vi "env-toolkit-ui.vi"() -> ()   [LabVIEW 2025]
doc: "Environment Toolkit for TestStand - Graphical User Interface"
uses:
  TSDiscovery/TSDiscovery.lvclass
  C:/Users/juanj/Documents/hasbun_wood_engineering/github/Environment-Toolkit-for-TestStand/src/TSDiscovery/TSDiscovery.lvclass
  C:/Users/juanj/Documents/hasbun_wood_engineering/github/Environment-Toolkit-for-TestStand/src/ITSDiscovery/ITSDiscovery.lvclass
  TSDiscovery Mock/TSDiscovery Mock.lvclass
  C:/Users/juanj/Documents/hasbun_wood_engineering/github/Environment-Toolkit-for-TestStand/src/TSDiscovery Mock/TSDiscovery Mock.lvclass
  Process Executor/Process Executor.lvclass
  C:/Users/juanj/Documents/hasbun_wood_engineering/github/Environment-Toolkit-for-TestStand/src/Process Executor/Process Executor.lvclass
  C:/Users/juanj/Documents/hasbun_wood_engineering/github/Environment-Toolkit-for-TestStand/src/IProcess Executor/IProcess Executor.lvclass
  Type Definitions/UI State--enum.ctl
  Libraries/TS Environment Manager/TS Environment Manager.lvlib
  Type Definitions/UI Data--cluster.ctl
  Type Definitions/Architecture--enum.ctl
  Type Definitions/Profile--cluster.ctl
  Type Definitions/TSInstall--cluster.ctl
  <vilib>/Utility/miscctls.llb/LVRectTypeDef.ctl
  <vilib>/Utility/miscctls.llb/LVPointTypeDef.ctl
  Type Definitions/Progress Display--enum.ctl
  Type Definitions/Execution Plan--cluster.ctl
  <vilib>/Platform/browser.llb/Open URL in Default Browser (string).vi
  ITSDiscovery/ITSDiscovery.lvclass
  IProcess Executor/IProcess Executor.lvclass
panel:
  in  "Open":bool
  out "Progress Display String":string
  in  "License":bool
  in  "Clear Environment":bool
  in  "Progress Display":T1
  in  "New Profiles File":path
  in  "Environment (Profile Mgt)":path caption="Environment"
  out "Environment (Launch)":path caption="Environment"
  in  "Hyperlink HWE":bool
  in  "Third Party Licenses":bool
  in  "Launch":bool
  in  "Set File":bool
  in  "Delete Profile":bool
  in  "Add Profile":bool
  in  "New Profile Name":string
  in  "Profiles":i32(listbox)
  in  "Installations":i32(listbox)
  out "Profiles File":path
  # "Hidden elements"
  # "Profile Management"
  # "Launch"
  # "This software is released under the MIT License\nCopyright (c) 2026 Juan Jose Hasbun Wood"
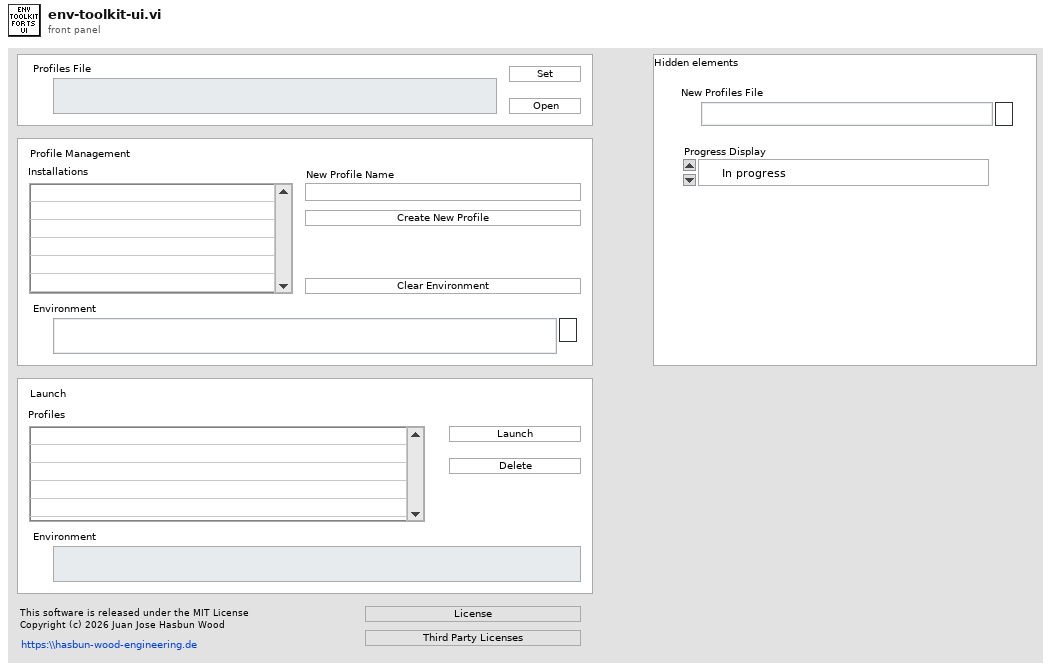
[diagram p1: front panel]
types:
  T1 = typedef "Progress Display--enum.ctl" = enum16{"     In progress", "     In progress.", "     In progress..", "     In progress..."}
  T2 = typedef "UI Data--cluster.ctl" = cluster{"Profiles":T3[], "Installations":T5[], "Event Structure Timeout":i32, "IProcess Executor.lvclass":refnum<class "IProcess Executor.lvclass">, "ITSDiscovery.lvclass":refnum<class "ITSDiscovery.lvclass">}
  T3 = typedef "Profile--cluster.ctl" = cluster{"Name":string, "Version":string, "Architecture":T4, "Environment":path}
  T4 = typedef "Architecture--enum.ctl" = enum16{"32bit", "64bit"}
  T5 = typedef "TSInstall--cluster.ctl" = cluster{"Version":string, "Architecture":T4, "Version Key":string, "ID":string}
  T6 = typedef "UI State--enum.ctl" = enum16{"Init", "Idle", "Add", "Delete", "Launch SeqEdit", "Error", "Exit", "License", "Update Profiles", "Update Installations", "Set File", "Start In Progress", "Stop In Progress", "Activate Version", "Third Party Licenses"}
  T7 = typedef "TS Environment Manager.lvlib/Broadcast Events--cluster.ctl" = cluster{"Module Did Init":refnum<user-event>, "Status Updated":refnum<user-event>, "Error Reported":refnum<user-event>, "Module Did Stop":refnum<user-event>, "Update Module Execution Status":refnum<user-event>, "Version Activated":refnum<user-event>, "Launched SeqEdit":refnum<user-event>}
  T8 = typedef "LVPointTypeDef.ctl" = cluster{"Horizontal":i16, "Vertical":i16}
  T9 = typedef "Execution Plan--cluster.ctl" = cluster{"Exe Path":path, "Args":string[], "Timeout":i32}
  T10 = typedef "LVRectTypeDef.ctl" = cluster{"Left":i16, "Top":i16, "Right":i16, "Bottom":i16}
  T11 = enum8{"Enabled", "Disabled", "Disabled and Grayed Out"}
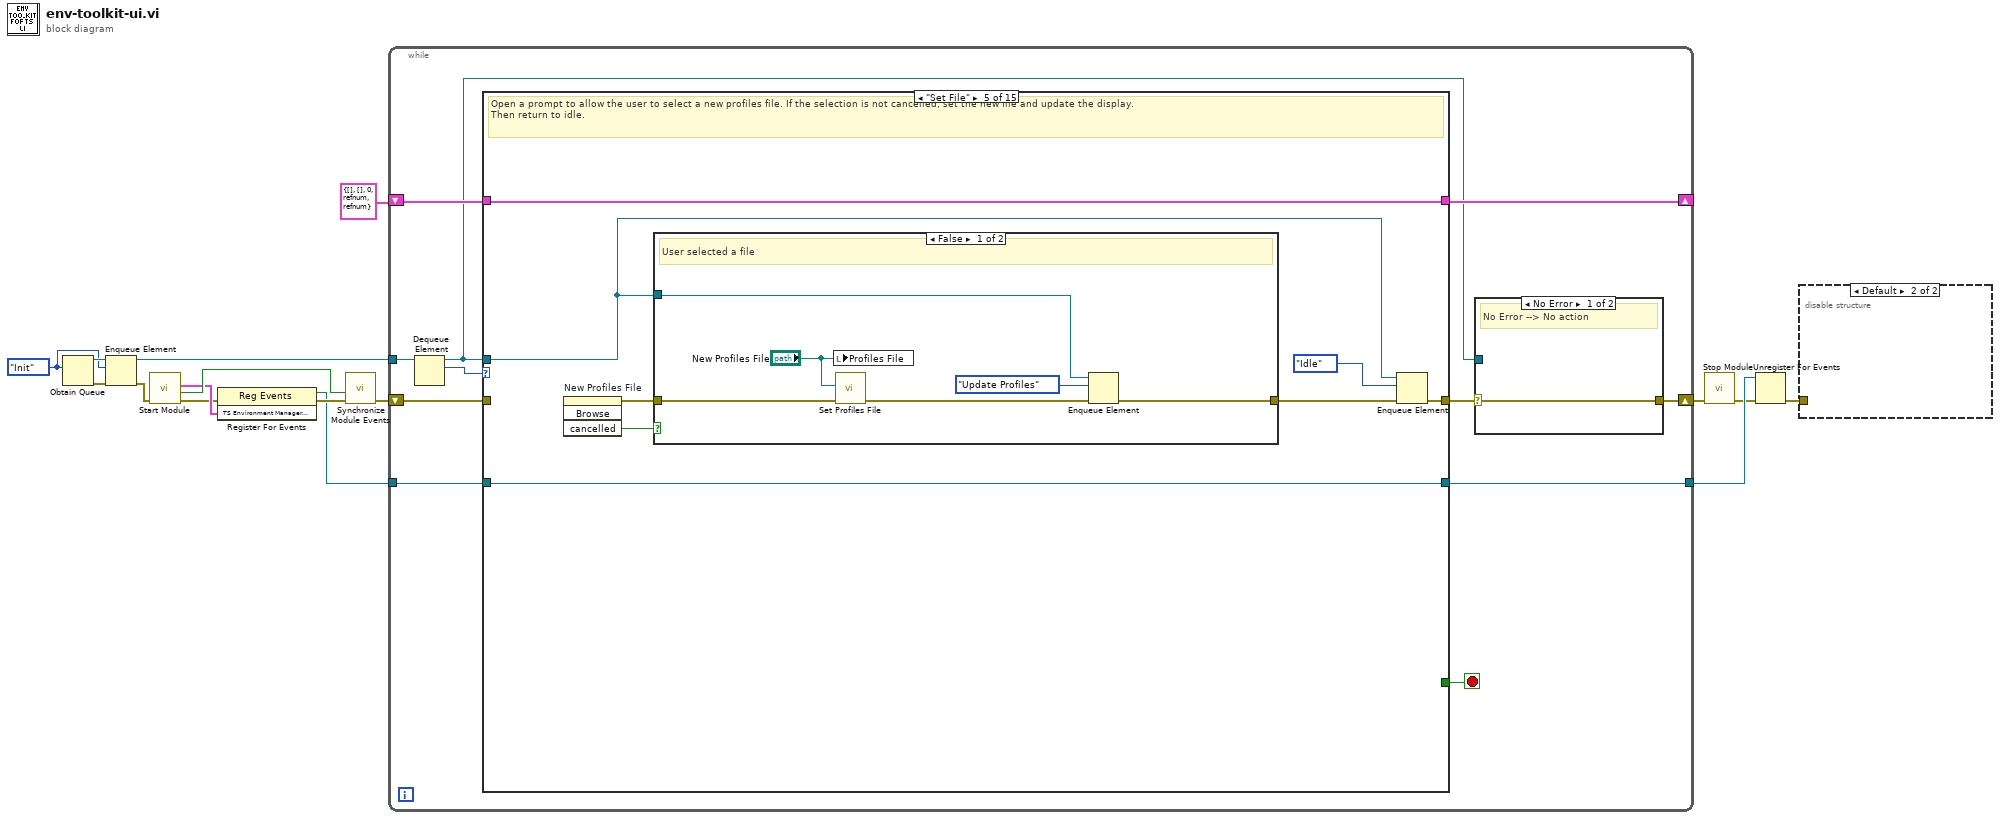
[diagram p0: block diagram]
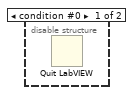
[diagram p2: hidden frame]
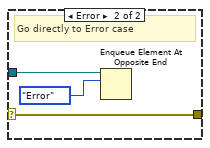
[diagram p3: hidden frame]
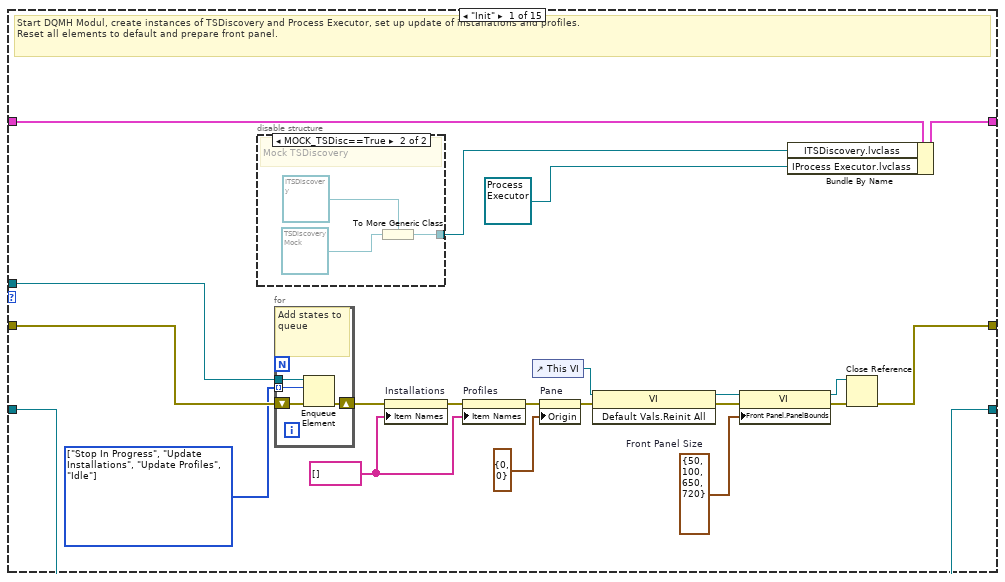
[diagram p4: hidden frame]
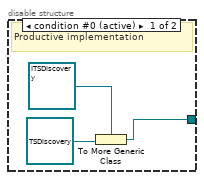
[diagram p5: hidden frame]
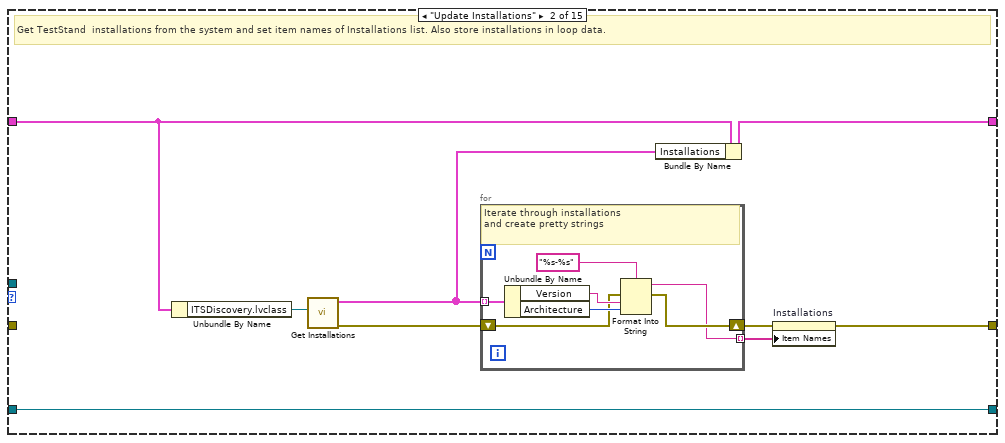
[diagram p6: hidden frame]
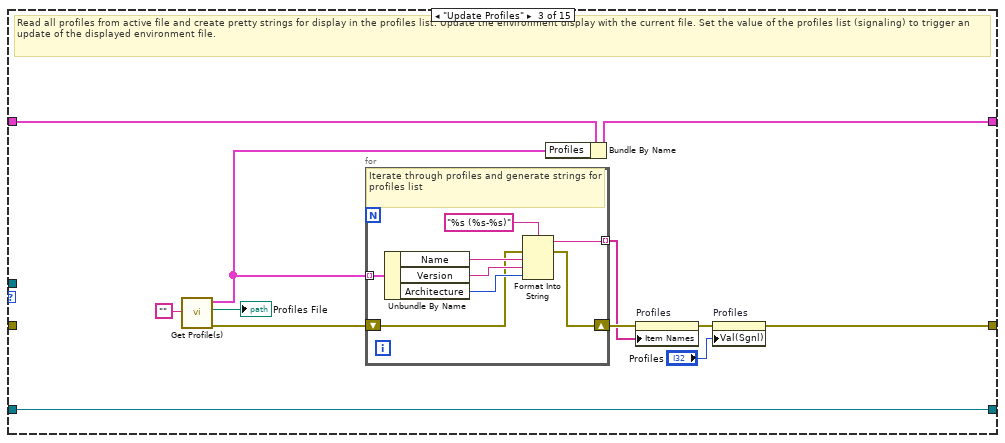
[diagram p7: hidden frame]
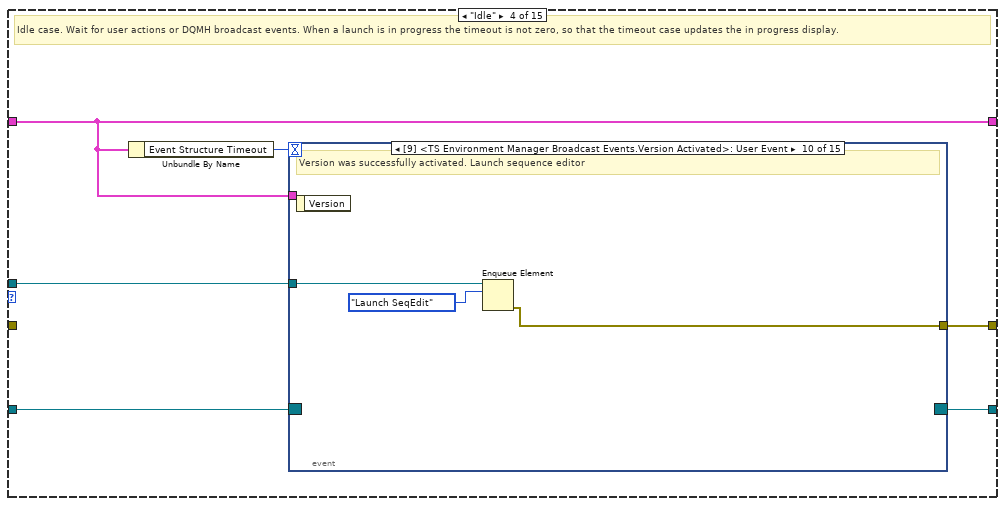
[diagram p8: hidden frame]
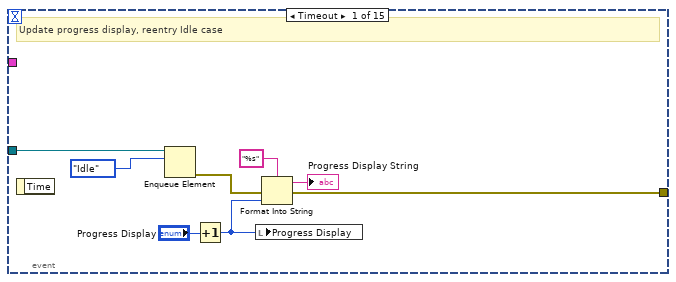
[diagram p9: hidden frame]
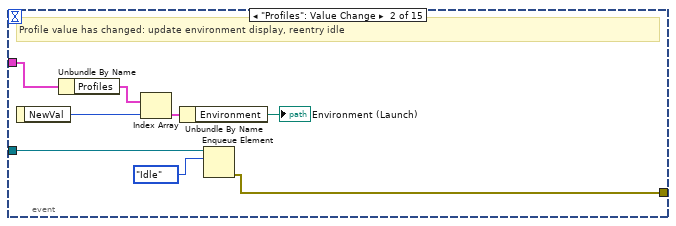
[diagram p10: hidden frame]
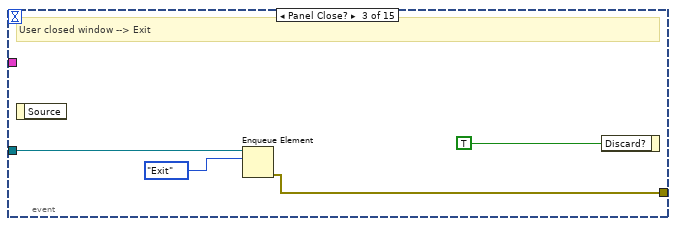
[diagram p11: hidden frame]
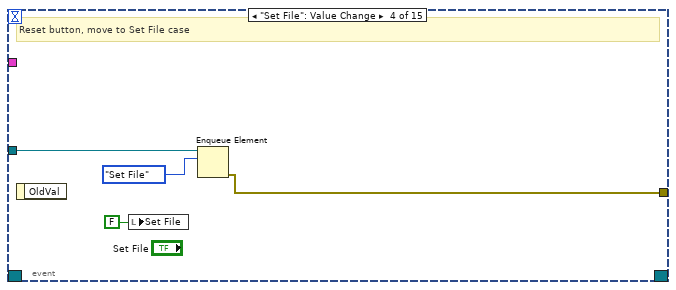
[diagram p12: hidden frame]
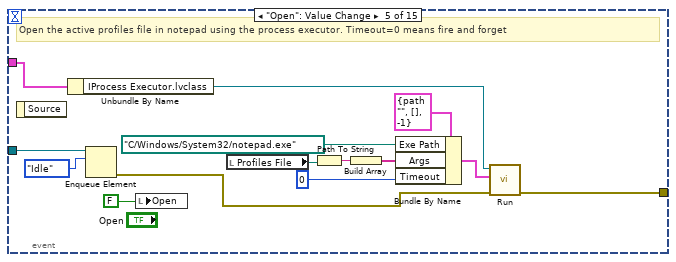
[diagram p13: hidden frame]
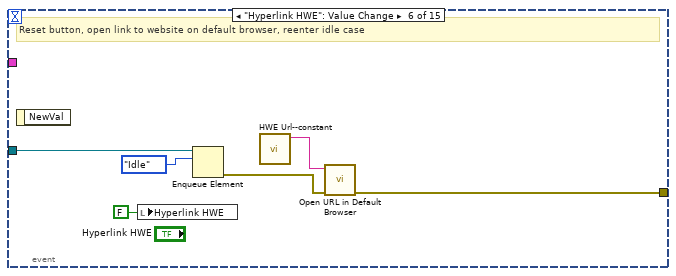
[diagram p14: hidden frame]
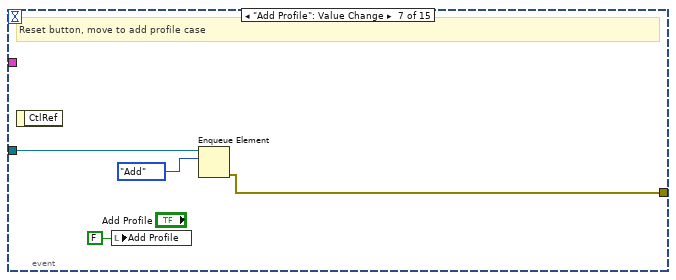
[diagram p15: hidden frame]
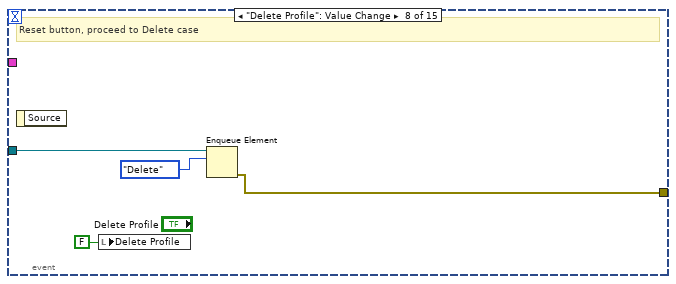
[diagram p16: hidden frame]
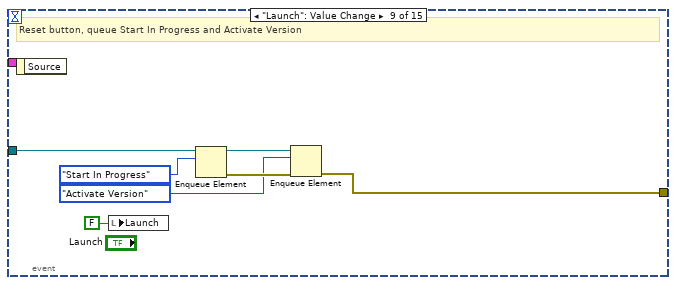
[diagram p17: hidden frame]
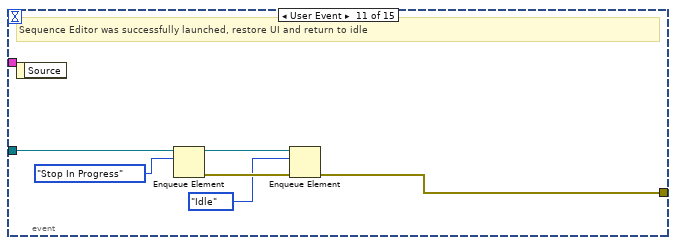
[diagram p18: hidden frame]
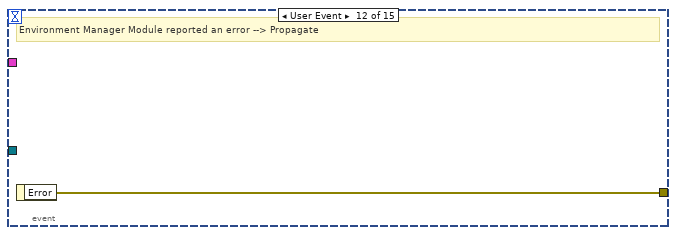
[diagram p19: hidden frame]
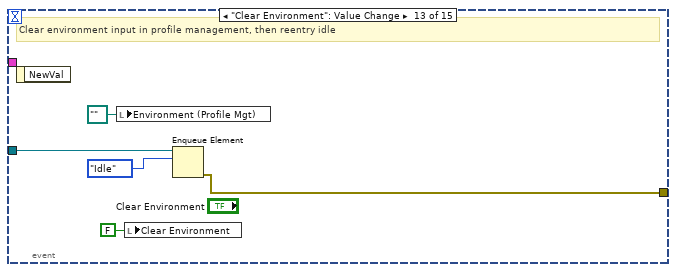
[diagram p20: hidden frame]
diagram:
  w14 = UI_State--enum."Init"
  n1 = Obtain Queue(element data type=w14) -> (queue out=w16:refnum<queue>, error out=w15:errorcluster)  [unwired: 4 in, 1 out]
  n2 = Enqueue Element(queue=w16, element=w14, error in (no error)=w15) -> (queue out=w13:refnum<queue>, error out=w7:errorcluster)  [unwired: 1 in, 1 out]
  n3 = call "Start Module.vi"("error in"=w7) -> ("error out"=w9:errorcluster, "Wait for Event Sync?"=w11:bool, "TS Environment Manager Broadcast Events"=w10:T7)  [unwired: 6 in, 2 out]
  n4 = register-events(error in=w9, w10) -> (reference out=w5:refnum<event-registration>, error out=w8:errorcluster)  [unwired: 1 in]
  n5 = call "Synchronize Module Events.vi"("error in"=w8, "Wait for Event Sync?"=w11) -> ("error out"=w6:errorcluster)  [unwired: 9 in]
  n6 = while {
    tunnel: w13 -> [w27]
    shift-right: [w22] -> w2
    shift-left: w6 -> [w17]
    shift-right: [w24] -> _
    shift-left: T2 {"Profiles"=[], "Installations"=[], "Event Structure Timeout"=0, "IProcess Executor.lvclass"=refnum, "ITSDiscovery.lvclass"=refnum} ("UI Data") -> [w25]
    tunnel: w5 -> [w19]
    tunnel: [w18] -> w3
    stop <- w20 stop-if-true
    n7 = Dequeue Element(queue=w27) -> (queue out=w21:refnum<queue>, element=w26:T6)  [unwired: 2 in, 2 out]
    n8 = case shown="\"Set File\"" w26 {
      tunnel: w21 -> [w49 _ _ w104 w190 w208 _ w235 w252 w262 w280 w294 w304 _ _]
      tunnel: w17 -> [w48 _ _ _ _ w205 _ _ _ _ _ _ _ _ _]
      tunnel: w25 -> [w52 w65 w85 w99 w187 w202 w219 w225 w242 w272 w286 w297 w314 w325 w347]
      tunnel: [w50 w66 w86 w99 w187 w202 w219 w225 w242 w272 w286 w297 w314 w326 w348] -> w24
      tunnel: [w32 w67 w81 w103 w191 w207 w216 w222 w237 w255 w278 w295 w308 w327 w349] -> w23
      tunnel: [_ _ _ _ _ _ TRUE _ _ _ _ _ _ _ _] -> w20
      tunnel: w19 -> [w34 w63 w79 w102 w188 w206 w218 w236 w253 w259 w277 w291 w305 w323 w345]
      tunnel: [w34 w63 w79 w100 w188 w206 w218 w236 w253 w259 w277 w291 w305 w323 w345] -> w18
      frame "Init" {
        w41 = T10 {"Left"=50, "Top"=100, "Right"=650, "Bottom"=720}  # Front Panel Size
        w45 = string[] [] ("Item Names")
        w47 = T6[] [enum."Stop In Progress", enum."Update Installations", enum."Update Profiles", enum."Idle"] items=["Init", "Idle", "Add", "Delete", "Launch SeqEdit", "Error", "Exit", "License", "Update Profiles", "Update Installations", "Set File", "Start In Progress", "Stop In Progress", "Activate Version", "Third Party Licenses"]
        # "Start DQMH Modul, create instances of TSDiscovery and Process Executor, set up update of installations and profiles.\nReset all elements to default and prepare front panel."
        n9 = disable-structure shown="MOCK_TSDisc==True" {
          disable-tunnel: [w53 w56] -> w33
          frame condition #0 (active) {
            # "Productive implementation"
            n10 = To More Generic Class(target class=refnum<class "ITSDiscovery.lvclass"> refnum ("ITSDiscovery.lvclass"), reference=refnum<class "TSDiscovery.lvclass"> refnum ("TSDiscovery.lvclass")) -> (generic class reference=w53:refnum<class "ITSDiscovery.lvclass">)
          }
          frame condition #1 {
            # "Mock TSDiscovery"
            n11 = To More Generic Class(target class=refnum<class "ITSDiscovery.lvclass"> refnum ("ITSDiscovery.lvclass"), reference=refnum<class "TSDiscovery Mock.lvclass"> refnum ("TSDiscovery Mock.lvclass")) -> (generic class reference=w56:refnum<class "ITSDiscovery.lvclass">)
          }
        }
        n12 = for {
          tunnel: w49 -> [w62]
          tunnel: w47 -> [w60] mode=indexing
          shift-right: [w59] -> w36
          shift-left: w48 -> [w61]
          # "Add states to queue"
          n13 = Enqueue Element(queue=w62, element=w60, error in (no error)=w61) -> (error out=w59:errorcluster)  [unwired: 1 in, 2 out]
        }
        n14 = property on="Installations" class="LstBox (strict)"(error in=w36, "Item Names"=w45) -> (error out=w46:errorcluster)  [unwired: 1 in, 1 out]
        n15 = property on="Profiles" class="LstBox (strict)"(error in=w46, "Item Names"=w45) -> (error out=w44:errorcluster)  [unwired: 1 in, 1 out]
        n16 = control-ref of="This VI"() -> (w42:refnum<vi>)
        n17 = property on="Pane" class="Pane"(error in=w44, "Origin"=T8 {"Horizontal"=0, "Vertical"=0}) -> (error out=w43:errorcluster)  [unwired: 1 in, 1 out]
        n18 = invoke on="Invoke Node" class="VI" method="Default Vals.Reinit All"(reference=w42, error in=w43) -> (reference out=w40:refnum<vi>, error out=w39:errorcluster)  [unwired: 1 in, 1 out]
        n19 = property on="Property Node" class="VI"(reference=w40, error in=w39, "Front Panel.PanelBounds"=w41) -> (reference out=w38:refnum<vi>, error out=w37:errorcluster)
        n20 = Bundle By Name(cluster=w52, "ITSDiscovery.lvclass"=w33, "IProcess Executor.lvclass"=refnum<class "Process Executor.lvclass"> refnum ("Process Executor.lvclass")) -> (w50:T2)
        n21 = Close Reference(reference=w38, error in (no error)=w37) -> (error out=w32:errorcluster)
      }
      frame "Update Installations" {
        # "Get TestStand  installations from the system and set item names of Installations list. Also store installations in loop data."
        n22 = Unbundle By Name(w65) -> ("ITSDiscovery.lvclass"=w68:refnum<class "ITSDiscovery.lvclass">)
        n23 = call "Get Installations.vi"("ITSDiscovery.lvclass"=w68) -> ("error out"=w71:errorcluster, "Installations"=w64:T5[])  [unwired: 8 in, 1 out]
        n24 = for {
          tunnel: w64 -> [w78] mode=indexing
          shift-right: [w73] -> w69
          shift-left: w71 -> [w74]
          tunnel: [w72] -> w70 mode=indexing
          # "Iterate through installations\nand create pretty strings"
          n25 = Unbundle By Name(w78) -> ("Version"=w76:string, "Architecture"=w75:T4)
          n26 = Format Into String(format string="%s-%s", error in=w74, w76, w75) -> (resulting string=w72:string, error out=w73:errorcluster)  [unwired: 1 in]
        }
        n27 = Bundle By Name(cluster=w65, "Installations"=w64) -> (w66:T2)
        n28 = property on="Installations" class="LstBox (strict)"(error in=w69, "Item Names"=w70) -> (error out=w67:errorcluster)  [unwired: 1 in, 1 out]
      }
      frame "Update Profiles" {
        # "Read all profiles from active file and create pretty strings for display in the profiles list. Update the environment display with the current file. Set the value of the profiles list (signaling) to trigger an update of the displayed environment file."
        n29 = call "Get Profile(s).vi"("Name"="" ("Empty String Constant")) -> ("error out"=w89:errorcluster, "File"=→"Profiles File":path, "Profile(s)"=w84:T3[])  [unwired: 7 in, 1 out]
        n30 = for {
          tunnel: w84 -> [w98] mode=indexing
          shift-right: [w92] -> w88
          shift-left: w89 -> [w93]
          tunnel: [w91] -> w87 mode=indexing
          # "Iterate through profiles and generate strings for profiles list"
          n31 = Unbundle By Name(w98) -> ("Name"=w96:string, "Version"=w95:string, "Architecture"=w94:T4)
          n32 = Format Into String(format string="%s (%s-%s)", error in=w93, w96, w95, w94) -> (resulting string=w91:string, error out=w92:errorcluster)  [unwired: 1 in]
        }
        n33 = Bundle By Name(cluster=w85, "Profiles"=w84) -> (w86:T2)
        n34 = property on="Profiles" class="LstBox (strict)"(error in=w88, "Item Names"=w87) -> (error out=w82:errorcluster)  [unwired: 1 in, 1 out]
        n35 = property on="Profiles" class="LstBox (strict)"(error in=w82, "Val(Sgnl)"="Profiles") -> (error out=w81:errorcluster)  [unwired: 1 in, 1 out]
      }
      frame "Idle" {
        # "Idle case. Wait for user actions or DQMH broadcast events. When a launch is in progress the timeout is not zero, so that the timeout case updates the in progress display."
        n36 = Unbundle By Name(w99) -> ("Event Structure Timeout"=w101:i32)
        n37 = event shown="[9] <TS Environment Manager Broadcast Events.Version Activated>: User Event" {
          selector: w102 -> [_ _ _ _ _ _ _ _ _ _ _ _ _ _ _]
          dyn-events: [_ _ _ _ _ _ _ _ _ _ _ _ _ _ _] -> w100
          timeout: w101 -> [_ _ _ _ _ _ _ _ _ _ _ _ _ _ _]
          tunnel: w99 -> [_ w113 _ _ w129 _ _ _ _ _ _ _ _ _ _]
          tunnel: w104 -> [w107 w116 w123 w128 w141 w145 w152 w156 w162 w166 w172 _ w176 w181 w186]
          tunnel: [w108 w115 w121 w126 w131 w147 w151 w155 w160 w165 w170 w173 w174 w180 w185] -> w103
          event Timeout {
            # "Update progress display, reentry Idle case"
            n38 = event-data() -> ()  [unwired: 1 in, 1 out]
            n39 = Enqueue Element(queue=w107, element=UI_State--enum."Idle") -> (error out=w105:errorcluster)  [unwired: 2 in, 2 out]
            n40 = Increment(x="Progress Display") -> (x+1=w111:T1)
            n41 = local write "Progress Display"(w111) -> ()
            n42 = Format Into String(format string="%s", error in=w105, w111) -> (resulting string=→"Progress Display String":string, error out=w108:errorcluster)  [unwired: 1 in]
          }
          event "Profiles": Value Change {
            # "Profile value has changed: update environment display, reentry idle"
            n43 = event-data() -> ("NewVal"=w119:i32)  [unwired: 1 in]
            n44 = Unbundle By Name(w113) -> ("Profiles"=w120:T3[])
            n45 = Index Array(array=w120, index=w119) -> (element=w118:T3)
            n46 = Unbundle By Name(w118) -> ("Environment"=→"Environment (Launch)":path)
            n47 = Enqueue Element(queue=w116, element=UI_State--enum."Idle") -> (error out=w115:errorcluster)  [unwired: 2 in, 2 out]
          }
          event Panel Close? {
            # "User closed window --> Exit"
            n48 = event-data() -> ()  [unwired: 1 in, 1 out]
            n49 = Enqueue Element(queue=w123, element=UI_State--enum."Exit") -> (error out=w121:errorcluster)  [unwired: 2 in, 2 out]
            n50 = event-data ("Event Filter Node")("Discard?"=TRUE) -> ()  [unwired: 1 in, 1 out]
          }
          event "Set File": Value Change {
            # "Reset button, move to Set File case"
            n51 = event-data() -> ()  [unwired: 1 in, 1 out]
            n52 = local write "Set File"(FALSE ("Set File")) -> ()
            n53 = Enqueue Element(queue=w128, element=UI_State--enum."Set File") -> (error out=w126:errorcluster)  [unwired: 2 in, 2 out]
          }
          event "Open": Value Change {
            # "Open the active profiles file in notepad using the process executor. Timeout=0 means fire and forget"
            n54 = event-data() -> ()  [unwired: 1 in, 1 out]
            n55 = Unbundle By Name(w129) -> ("IProcess Executor.lvclass"=w133:refnum<class "IProcess Executor.lvclass">)
            n56 = Enqueue Element(queue=w141, element=UI_State--enum."Idle") -> (error out=w130:errorcluster)  [unwired: 2 in, 2 out]
            n57 = local write "Open"(FALSE ("Open")) -> ()
            n58 = local read "Profiles File"() -> (w137:path)
            n59 = Path To String(path=w137) -> (string=w136:string)
            n60 = Build Array(w136) -> (w135:string[])
            n61 = Bundle By Name(cluster=T9 {"Exe Path"=path "", "Args"=[], "Timeout"=-1} ("Execution Plan"), "Exe Path"=path "C:/Windows/System32/notepad.exe", "Args"=w135, "Timeout"=0) -> (w132:T9)
            n62 = call-dynamic "Run.vi"("error in"=w130, "Execution Plan"=w132, "IProcess Executor in"=w133) -> ("error out"=w131:errorcluster)  [unwired: 7 in, 1 out]
          }
          event "Hyperlink HWE": Value Change {
            # "Reset button, open link to website on default browser, reenter idle case"
            n63 = event-data() -> ()  [unwired: 1 in, 1 out]
            n64 = local write "Hyperlink HWE"(FALSE ("Hyperlink HWE")) -> ()
            n65 = Enqueue Element(queue=w145, element=UI_State--enum."Idle") -> (error out=w143:errorcluster)  [unwired: 2 in, 2 out]
            n66 = call "HWE Url--constant.vi"() -> ("url"=w148:string)  [unwired: 11 in]
            n67 = call-poly <vilib>:"Open URL in Default Browser.vi"("error in (no error)"=w143, "URL"=w148) -> ("error out"=w147:errorcluster)  [unwired: 4 in, 1 out]
          }
          event "Add Profile": Value Change {
            # "Reset button, move to add profile case"
            n68 = event-data() -> ()  [unwired: 1 in, 1 out]
            n69 = local write "Add Profile"(FALSE ("Add Profile")) -> ()
            n70 = Enqueue Element(queue=w152, element=UI_State--enum."Add") -> (error out=w151:errorcluster)  [unwired: 2 in, 2 out]
          }
          event "Delete Profile": Value Change {
            # "Reset button, proceed to Delete case"
            n71 = event-data() -> ()  [unwired: 1 in, 1 out]
            n72 = local write "Delete Profile"(FALSE ("Delete Profile")) -> ()
            n73 = Enqueue Element(queue=w156, element=UI_State--enum."Delete") -> (error out=w155:errorcluster)  [unwired: 2 in, 2 out]
          }
          event "Launch": Value Change {
            # "Reset button, queue Start In Progress and Activate Version"
            n74 = event-data() -> ()  [unwired: 1 in, 1 out]
            n75 = local write "Launch"(FALSE ("Launch")) -> ()
            n76 = Enqueue Element(queue=w162, element=UI_State--enum."Start In Progress") -> (queue out=w157:refnum<queue>, error out=w159:errorcluster)  [unwired: 2 in, 1 out]
            n77 = Enqueue Element(queue=w157, element=UI_State--enum."Activate Version", error in (no error)=w159) -> (error out=w160:errorcluster)  [unwired: 1 in, 2 out]
          }
          event User Event {
            # "Version was successfully activated. Launch sequence editor"
            n78 = event-data() -> ()  [unwired: 1 in, 1 out]
            n79 = Enqueue Element(queue=w166, element=UI_State--enum."Launch SeqEdit") -> (error out=w165:errorcluster)  [unwired: 2 in, 2 out]
          }
          event User Event {
            # "Sequence Editor was successfully launched, restore UI and return to idle"
            n80 = event-data() -> ()  [unwired: 1 in, 1 out]
            n81 = Enqueue Element(queue=w172, element=UI_State--enum."Stop In Progress") -> (queue out=w169:refnum<queue>, error out=w171:errorcluster)  [unwired: 2 in, 1 out]
            n82 = Enqueue Element(queue=w169, element=UI_State--enum."Idle", error in (no error)=w171) -> (error out=w170:errorcluster)  [unwired: 1 in, 2 out]
          }
          event User Event {
            # "Environment Manager Module reported an error --> Propagate"
            n83 = event-data() -> ("Error"=w173:errorcluster)  [unwired: 1 in]
          }
          event "Clear Environment": Value Change {
            # "Clear environment input in profile management, then reentry idle"
            n84 = event-data() -> ()  [unwired: 1 in, 1 out]
            n85 = local write "Environment (Profile Mgt)"(path "" ("Environment (Profile Mgt)")) -> ()
            n86 = local write "Clear Environment"(FALSE ("Clear Environment")) -> ()
            n87 = Enqueue Element(queue=w176, element=UI_State--enum."Idle") -> (error out=w174:errorcluster)  [unwired: 2 in, 2 out]
          }
          event "Third Party Licenses": Value Change {
            # "Display third party licenses"
            n88 = event-data() -> ()  [unwired: 1 in, 1 out]
            n89 = local write "Third Party Licenses"(FALSE ("License Info")) -> ()
            n90 = Enqueue Element(queue=w181, element=UI_State--enum."Third Party Licenses") -> (error out=w180:errorcluster)  [unwired: 2 in, 2 out]
          }
          event "License": Value Change {
            # "Display license"
            n91 = event-data() -> ()  [unwired: 1 in, 1 out]
            n92 = local write "License"(FALSE ("License")) -> ()
            n93 = Enqueue Element(queue=w186, element=UI_State--enum."License") -> (error out=w185:errorcluster)  [unwired: 2 in, 2 out]
          }
        }
      }
      frame "Set File" {
        # "Open a prompt to allow the user to select a new profiles file. If the selection is not cancelled, set the new file and update the display.\nThen return to idle."
        n94 = invoke on="New Profiles File" class="Path" method="Browse"() -> (error out=w193:errorcluster, "cancelled"=w194:bool)  [unwired: 4 in, 2 out]
        n95 = case shown="False" w194 {
          tunnel: [w197 w201] -> w192
          tunnel: w193 -> [w200 w201]
          tunnel: w190 -> [w196 _]
          frame False {
            # "User selected a file"
            n96 = local write "Profiles File"("New Profiles File") -> ()
            n97 = call "Set Profiles File.vi"("error in"=w200, "File Path"="New Profiles File") -> ("error out"=w198:errorcluster)  [unwired: 9 in]
            n98 = Enqueue Element(queue=w196, element=UI_State--enum."Update Profiles", error in (no error)=w198) -> (error out=w197:errorcluster)  [unwired: 1 in, 2 out]
          }
          frame True {
            # "User cancelled prompt"
          }
        }
        n99 = Enqueue Element(queue=w190, element=UI_State--enum."Idle", error in (no error)=w192) -> (error out=w191:errorcluster)  [unwired: 1 in, 2 out]
      }
      frame "Error" {
        # "Display error message. For selected error codes continue operation, for any other stop application (go back to idle)."
        n100 = Unbundle By Name(w205) -> ("code"=w204:i32)
        n101 = call <vilib>:"Simple Error Handler.vi"("error in (no error)"=w205) -> ("error out"=w212:errorcluster)  [unwired: 4 in, 4 out]
        n102 = case shown="Default" w204 {
          tunnel: [UI_State--enum."Exit" ("element") UI_State--enum."Idle" ("element")] -> w203
          frame Default {
            # "Other errors --> Exit"
          }
          frame 510006, 510008, 510014 {
            # "Minor errors"
          }
        }
        n103 = call <vilib>:"Clear Errors.vi"("error in (no error)"=w212) -> ("error out"=w211:errorcluster)  [unwired: 5 in, 1 out]
        n104 = Flush Queue(queue=w208, error in (no error)=w211) -> (queue out=w209:refnum<queue>, error out=w210:errorcluster)  [unwired: 1 out]
        n105 = Enqueue Element(queue=w209, element=w203, error in (no error)=w210) -> (error out=w207:errorcluster)  [unwired: 1 in, 2 out]
      }
      frame "Exit" {
        w215 = string[] [] ("Item Names")
        # "Clean lists so that they are saved empty after execution from\ndevelopment environment"
        # "Stop loop"
        n106 = property on="Installations" class="LstBox (strict)"("Item Names"=w215) -> (error out=w217:errorcluster)  [unwired: 2 in, 1 out]
        n107 = property on="Profiles" class="LstBox (strict)"(error in=w217, "Item Names"=w215) -> (error out=w216:errorcluster)  [unwired: 1 in, 1 out]
      }
      frame "License" {
        # "Open LICENSE file in text editor, then return to idle. The file must be in the same folder as the exe."
        n108 = Enqueue Element(queue=w235, element=UI_State--enum."Idle") -> (error out=w221:errorcluster)  [unwired: 2 in, 2 out]
        n109 = Unbundle By Name(w225) -> ("IProcess Executor.lvclass"=w224:refnum<class "IProcess Executor.lvclass">)
        n110 = call <vilib>:"Application Directory.vi"() -> ("Application Directory"=w232:path)
        n111 = Build Path(base path=w232, name or relative path=path "LICENSE") -> (appended path=w226:path)
        n112 = Path To String(path=w226) -> (string=w229:string)
        n113 = call "Text Editor Path--constant.vi"() -> ("Path"=w228:path)  [unwired: 11 in]
        n114 = Build Array(w229) -> (w230:string[])
        n115 = Bundle By Name(cluster=T9 {"Exe Path"=path "", "Args"=[], "Timeout"=-1} ("Execution Plan"), "Exe Path"=w228, "Args"=w230, "Timeout"=-1) -> (w223:T9)
        n116 = call-dynamic "Run.vi"("error in"=w221, "Execution Plan"=w223, "IProcess Executor in"=w224) -> ("error out"=w222:errorcluster)  [unwired: 7 in, 1 out]
      }
      frame "Third Party Licenses" {
        # "Open THIRD_PARTY_LICENSES file in text editor, then the DQMH about window, then return to idle. The file must be in the same folder as the exe."
        n117 = Enqueue Element(queue=w252, element=UI_State--enum."Idle") -> (error out=w239:errorcluster)  [unwired: 2 in, 2 out]
        n118 = Unbundle By Name(w242) -> ("IProcess Executor.lvclass"=w241:refnum<class "IProcess Executor.lvclass">)
        n119 = call <vilib>:"Application Directory.vi"() -> ("Application Directory"=w249:path)
        n120 = Build Path(base path=w249, name or relative path=path "THIRD_PARTY_LICENSES") -> (appended path=w243:path)
        n121 = Path To String(path=w243) -> (string=w246:string)
        n122 = call "Text Editor Path--constant.vi"() -> ("Path"=w245:path)  [unwired: 11 in]
        n123 = Build Array(w246) -> (w247:string[])
        n124 = Bundle By Name(cluster=T9 {"Exe Path"=path "", "Args"=[], "Timeout"=-1} ("Execution Plan"), "Exe Path"=w245, "Args"=w247, "Timeout"=-1) -> (w240:T9)
        n125 = call-dynamic "Run.vi"("error in"=w239, "Execution Plan"=w240, "IProcess Executor in"=w241) -> ("error out"=w238:errorcluster)  [unwired: 7 in, 1 out]
        n126 = call <vilib>:"DQMH_About Box.vi"("error in"=w238) -> ("error out"=w237:errorcluster)  [unwired: 10 in]
      }
      frame "Add" {
        w260 = T6[] [enum."Update Profiles", enum."Idle"] items=["Init", "Idle", "Add", "Delete", "Launch SeqEdit", "Error", "Exit", "License", "Update Profiles", "Update Installations", "Set File", "Start In Progress", "Stop In Progress", "Activate Version", "Third Party Licenses"]
        # "Clear profile name"
        # "Create a new profile using parameters from UI, reset relevant user inputs and then proceed to update profiles and back to idle"
        n127 = Unbundle By Name(w272) -> ("Installations"=w271:T5[])
        n128 = for {
          tunnel: w262 -> [w276]
          tunnel: w260 -> [w274] mode=indexing
          shift-right: [w273] -> w261
          shift-left: _ -> [w275]
          # "Add states to queue"
          n129 = Enqueue Element(queue=w276, element=w274, error in (no error)=w275) -> (error out=w273:errorcluster)  [unwired: 1 in, 2 out]
        }
        n130 = Index Array(array=w271, index="Installations") -> (element=w267:T5)
        n131 = Unbundle By Name(w267) -> ("Version"=w266:string, "Architecture"=w265:T4)
        n132 = Bundle By Name(cluster=T3 {"Name"="", "Version"="", "Architecture"=enum."32bit", "Environment"=path ""} ("Profile"), "Name"="New Profile Name", "Version"=w266, "Architecture"=w265, "Environment"="Environment (Profile Mgt)") -> (w263:T3)
        n133 = call "Add Profile.vi"("error in"=w261, "Profile"=w263) -> ("error out"=w258:errorcluster)  [unwired: 8 in, 1 out]
        n134 = property on="New Profile Name" class="Str"(error in=w258, "Value"="") -> (error out=w256:errorcluster)  [unwired: 1 in, 1 out]
        n135 = property on="Environment (Profile Mgt)" class="Path"(error in=w256, "Value"=path "") -> (error out=w255:errorcluster)  [unwired: 1 in, 1 out]
      }
      frame "Delete" {
        w281 = T6[] [enum."Update Profiles", enum."Idle"] items=["Init", "Idle", "Add", "Delete", "Launch SeqEdit", "Error", "Exit", "License", "Update Profiles", "Update Installations", "Set File", "Start In Progress", "Stop In Progress", "Activate Version", "Third Party Licenses"]
        # "Delete currently selected profile in Profiles list, proceed to update profiles and back to idle."
        n136 = for {
          tunnel: w280 -> [w290]
          tunnel: w281 -> [w288] mode=indexing
          shift-right: [w287] -> w279
          shift-left: _ -> [w289]
          # "Add states to queue"
          n137 = Enqueue Element(queue=w290, element=w288, error in (no error)=w289) -> (error out=w287:errorcluster)  [unwired: 1 in, 2 out]
        }
        n138 = Unbundle By Name(w286) -> ("Profiles"=w285:T3[])
        n139 = local read "Profiles"() -> (w284:i32)
        n140 = Index Array(array=w285, index=w284) -> (element=w283:T3)
        n141 = Unbundle By Name(w283) -> ("Name"=w282:string)
        n142 = call "Delete Profile.vi"("error in"=w279, "Name"=w282) -> ("error out"=w278:errorcluster)  [unwired: 8 in, 1 out]
      }
      frame "Activate Version" {
        # "Run Activate Version request but do not wait for reply (so that the UI will not be blocked). Completion of activation will be received in Idle through the corresponding\nbroadcast event case."
        n143 = Enqueue Element(queue=w294, element=UI_State--enum."Idle") -> (error out=w292:errorcluster)  [unwired: 2 in, 2 out]
        n144 = Unbundle By Name(w297) -> ("ITSDiscovery.lvclass"=w298:refnum<class "ITSDiscovery.lvclass">, "IProcess Executor.lvclass"=w299:refnum<class "IProcess Executor.lvclass">, "Profiles"=w302:T3[])
        n145 = local read "Profiles"() -> (w301:i32)
        n146 = Index Array(array=w302, index=w301) -> (element=w300:T3)
        n147 = Unbundle By Name(w300) -> ("Version"=w303:string)
        n148 = call "Activate Version.vi"("wait for reply (T)"=FALSE, "ITSDiscovery.lvclass"=w298, "error in"=w292, "IProcess Executor.lvclass"=w299, "Version"=w303) -> ("error out"=w295:errorcluster)  [unwired: 5 in, 1 out]
      }
      frame "Launch SeqEdit" {
        # "Run Launch Sequence Editor request but do not wait for reply (so that the UI will not be blocked). \nCompletion of launching will be received in Idle through the corresponding broadcast event case."
        n149 = Unbundle By Name(w314) -> ("ITSDiscovery.lvclass"=w311:refnum<class "ITSDiscovery.lvclass">, "IProcess Executor.lvclass"=w310:refnum<class "IProcess Executor.lvclass">, "Profiles"=w315:T3[])
        n150 = local read "Profiles"() -> (w313:i32)
        n151 = Enqueue Element(queue=w304, element=UI_State--enum."Idle") -> (error out=w307:errorcluster)  [unwired: 2 in, 2 out]
        n152 = Index Array(array=w315, index=w313) -> (element=w312:T3)
        n153 = Unbundle By Name(w312) -> ("Architecture"=w317:T4, "Version"=w318:string, "Environment"=w316:path)
        n154 = call "Launch Sequence Editor.vi"("Environment"=w316, "Architecture"=w317, "wait for reply (T)"=FALSE, "Version"=w318, "error in"=w307, "IProcess Executor.lvclass"=w310, "ITSDiscovery.lvclass"=w311) -> ("error out"=w308:errorcluster)  [unwired: 3 in, 1 out]
      }
      frame "Start In Progress" {
        w321 = T11."Disabled and Grayed Out" ("Disabled")
        # "Set timeout for idle event structure"
        # "Disable all elements, make progress display visible"
        n155 = property on="Profiles File" class="Path"("DisabledEnum"=w321) -> (error out=w337:errorcluster)  [unwired: 2 in, 1 out]
        n156 = property on="Set File" class="Bool (strict)"("DisabledEnum"=w321) -> (error out=w336:errorcluster)  [unwired: 2 in, 1 out]
        n157 = property on="Installations" class="LstBox (strict)"("DisabledEnum"=w321) -> (error out=w335:errorcluster)  [unwired: 2 in, 1 out]
        n158 = property on="New Profile Name" class="Str"("DisabledEnum"=w321) -> (error out=w334:errorcluster)  [unwired: 2 in, 1 out]
        n159 = property on="Add Profile" class="Bool (strict)"("DisabledEnum"=w321) -> (error out=w333:errorcluster)  [unwired: 2 in, 1 out]
        n160 = property on="Environment (Profile Mgt)" class="Path"("DisabledEnum"=w321) -> (error out=w332:errorcluster)  [unwired: 2 in, 1 out]
        n161 = property on="Profiles" class="LstBox (strict)"("DisabledEnum"=w321) -> (error out=w331:errorcluster)  [unwired: 2 in, 1 out]
        n162 = property on="Launch" class="Bool (strict)"("DisabledEnum"=w321) -> (error out=w330:errorcluster)  [unwired: 2 in, 1 out]
        n163 = property on="Delete Profile" class="Bool (strict)"("DisabledEnum"=w321) -> (error out=w329:errorcluster)  [unwired: 2 in, 1 out]
        n164 = property on="Environment (Launch)" class="Path"("DisabledEnum"=w321) -> (error out=w328:errorcluster)  [unwired: 2 in, 1 out]
        n165 = property on="Open" class="Bool (strict)"("DisabledEnum"=w321) -> (error out=w319:errorcluster)  [unwired: 2 in, 1 out]
        n166 = property on="Clear Environment" class="Bool (strict)"("DisabledEnum"=w321) -> (error out=w322:errorcluster)  [unwired: 2 in, 1 out]
        n167 = flat-sequence {
          tunnel: [w340] -> w320
          frame #0 {
            # "Reset progress display"
            n168 = local write "Progress Display"(Progress_Display--enum."     In progress" ("Progress Display")) -> ()
          }
          frame #1 {
            n169 = property on="Progress Display String" class="Str"("Visible"=TRUE) -> (error out=w340:errorcluster)  [unwired: 2 in, 1 out]
          }
        }
        n170 = Bundle By Name(cluster=w325, "Event Structure Timeout"=500) -> (w326:T2)
        n171 = Merge Errors(w337, w336, w335, w334, w333, w332, w331, w330, w329, w328, w322, w319, w320) -> (w327:errorcluster)
      }
      frame "Stop In Progress" {
        w343 = T11."Enabled" ("Disabled")
        # "Remove timeout for event structure"
        # "Enable all elements, make progress display invisible"
        n172 = property on="Open" class="Bool (strict)"("DisabledEnum"=w343) -> (error out=w341:errorcluster)  [unwired: 2 in, 1 out]
        n173 = property on="Profiles File" class="Path"("DisabledEnum"=w343) -> (error out=w359:errorcluster)  [unwired: 2 in, 1 out]
        n174 = property on="Set File" class="Bool (strict)"("DisabledEnum"=w343) -> (error out=w358:errorcluster)  [unwired: 2 in, 1 out]
        n175 = property on="Installations" class="LstBox (strict)"("DisabledEnum"=w343) -> (error out=w357:errorcluster)  [unwired: 2 in, 1 out]
        n176 = property on="New Profile Name" class="Str"("DisabledEnum"=w343) -> (error out=w356:errorcluster)  [unwired: 2 in, 1 out]
        n177 = property on="Add Profile" class="Bool (strict)"("DisabledEnum"=w343) -> (error out=w355:errorcluster)  [unwired: 2 in, 1 out]
        n178 = property on="Environment (Profile Mgt)" class="Path"("DisabledEnum"=w343) -> (error out=w354:errorcluster)  [unwired: 2 in, 1 out]
        n179 = property on="Profiles" class="LstBox (strict)"("DisabledEnum"=w343) -> (error out=w353:errorcluster)  [unwired: 2 in, 1 out]
        n180 = property on="Launch" class="Bool (strict)"("DisabledEnum"=w343) -> (error out=w352:errorcluster)  [unwired: 2 in, 1 out]
        n181 = property on="Delete Profile" class="Bool (strict)"("DisabledEnum"=w343) -> (error out=w351:errorcluster)  [unwired: 2 in, 1 out]
        n182 = property on="Environment (Launch)" class="Path"("DisabledEnum"=w343) -> (error out=w350:errorcluster)  [unwired: 2 in, 1 out]
        n183 = property on="Progress Display String" class="Str"("Visible"=FALSE) -> (error out=w342:errorcluster)  [unwired: 2 in, 1 out]
        n184 = property on="Clear Environment" class="Bool (strict)"("DisabledEnum"=w343) -> (error out=w344:errorcluster)  [unwired: 2 in, 1 out]
        n185 = Merge Errors(w359, w358, w357, w356, w355, w354, w353, w352, w351, w350, w344, w341, w342) -> (w349:errorcluster)
        n186 = Bundle By Name(cluster=w347, "Event Structure Timeout"=-1) -> (w348:T2)
      }
    }
    n187 = case shown="No Error" w23 {
      selector: w23 -> [w28 w29]
      tunnel: w21 -> [_ w31]
      tunnel: [w28 w29] -> w22
      frame No Error {
        # "No Error --> No action"
      }
      frame Error {
        # "Go directly to Error case"
        n188 = Enqueue Element At Opposite End(queue=w31, element=UI_State--enum."Error") -> ()  [unwired: 2 in, 3 out]
      }
    }
  }
  n189 = call "Stop Module.vi"("error in"=w2) -> ("error out"=w1:errorcluster)  [unwired: 10 in]
  n190 = Unregister For Events(event registration refnum=w3, error in=w1) -> (error out=w4:errorcluster)
  n191 = disable-structure "Conditional Disable Structure" shown="Default" {
    disable-tunnel: w4 -> [_ _]
    frame condition #0 {
      n192 = Quit LabVIEW() -> ()  [unwired: 1 in]
    }
    frame condition #1 (active) {
    }
  }
